vi "S2C_ExeScriptReset.vi"(8 "Error In":errorcluster, 11 "Script Data":string[][](array[string])) -> (0 "Error Out":errorcluster)   [LabVIEW 2015]
doc: "Loads script data into the executable table, and resets all cells to their default colors."
uses:
  Globals/S2C_Globals.vi
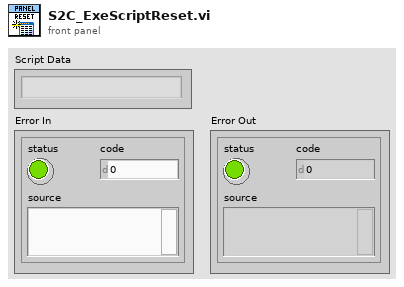
[diagram p1: front panel]
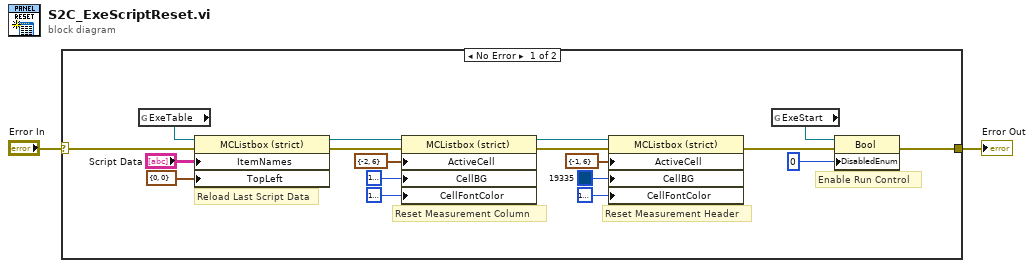
[diagram p0: block diagram]
diagram:
  n1 = case shown="No Error" "Error In" {
    selector: "Error In" -> [w12 w21]
    tunnel: [w3 w21] -> w1
    frame No Error {
      # "Enable Run Control"
      # "Reset Measurement Header"
      # "Reset Measurement Column"
      # "Reload Last Script Data"
      n2 = global read "S2C_Globals.vi" "ExeTable"() -> (w11:refnum<vi>)
      n3 = property on="Property Node" class="MCListbox (strict)"(reference=w11, error in=w12, "ItemNames"="Script Data", "TopLeft"=cluster{"Row":u32, "Column":u32} {"Row"=0, "Column"=0} ("Top Left Visible Cell")) -> (reference out=w9:refnum<vi>, error out=w14:errorcluster)
      n4 = property on="Property Node" class="MCListbox (strict)"(reference=w9, error in=w14, "ActiveCell"=cluster{"Row":i32, "Column":i32} {"Row"=-2, "Column"=6} ("Active Cell:Active Cell"), "CellBG"=u32 16777226, "CellFontColor"=u32 16777222) -> (reference out=w8:refnum<vi>, error out=w20:errorcluster)
      n5 = property on="Property Node" class="MCListbox (strict)"(reference=w8, error in=w20, "ActiveCell"=cluster{"Row":i32, "Column":i32} {"Row"=-1, "Column"=6} ("Active Cell:Active Cell"), "CellBG"=u32 19335, "CellFontColor"=u32 16777226) -> (error out=w6:errorcluster)  [unwired: 1 out]
      n6 = global read "S2C_Globals.vi" "ExeStart"() -> (w5:refnum<vi>)
      n7 = property class="Bool"(reference=w5, error in=w6, "DisabledEnum"=u8 0) -> (error out=w3:errorcluster)  [unwired: 1 out]
    }
    frame Error {
    }
  }
  "Error Out" <- w1
